vi "test-pose2d.vi"() -> ()   [LabVIEW 2019]
uses:
  <vilib>/Rock Robotics/WPI/ThirdParty/JAS_Junk/TrajLib/Translation_Equals.vi
  <vilib>/Rock Robotics/WPI/ThirdParty/JAS_Junk/TrajLib/Rotation_Equals.vi
  <vilib>/Rock Robotics/WPI/ThirdParty/JAS_Junk/TrajLib/Transform_Create_PosePose.vi
  <vilib>/Rock Robotics/WPI/ThirdParty/JAS_Junk/TrajLib/Pose_TransformBy.vi
  <vilib>/Rock Robotics/WPI/ThirdParty/JAS_Junk/TrajLib/Rotation_UnaryMinus.vi
  <vilib>/Rock Robotics/WPI/ThirdParty/JAS_Junk/TrajLib/Translation_RotateBy.vi
  <vilib>/Rock Robotics/WPI/ThirdParty/JAS_Junk/TrajLib/Translation_Minus.vi
  <vilib>/Rock Robotics/WPI/ThirdParty/JAS_Junk/TrajLib/Rotation_Minus.vi
  <vilib>/Rock Robotics/WPI/ThirdParty/JAS_Junk/TrajLib/Translation_Plus.vi
  <vilib>/Rock Robotics/WPI/ThirdParty/JAS_Junk/TrajLib/Rotation_Plus.vi
  <vilib>/Rock Robotics/WPI/ThirdParty/JAS_Junk/TrajLib/Rotation_RotateBy.vi
  <vilib>/Rock Robotics/WPI/ThirdParty/JAS_Junk/TrajLib/Rotation_CreateXY.vi
  <vilib>/Rock Robotics/WPI/ThirdParty/JAS_Junk/TrajLib/Util_CalcDist.vi
  <vilib>/Rock Robotics/WPI/ThirdParty/JAS_Junk/TrajLib/Trajectory_Library.lvlib
panel:
  out "T4 -- Deg -- 0":dbl
  out "T4 -- y -- 0":dbl
  out "T4 -- X -- 0":dbl
  out "T3 - False":bool
  out "T2 - True":bool
  out "T1 -- Deg -- 0":dbl
  out "T1 -- y -- 0":dbl
  out "T1 -- X -- 0":dbl
  out "T0 -- Deg -- 0":dbl
  out "T0 -- y -- 0":dbl
  out "T0 -- X -- 0":dbl
  # "Pose2D Test"
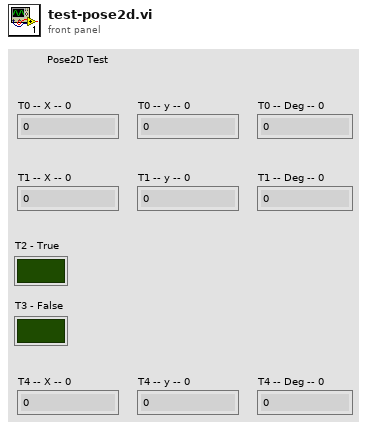
[diagram p1: front panel]
types:
  T1 = typedef "Trajectory_Library.lvlib/TRANSLATION2D.ctl" = cluster{"X":dbl, "Y":dbl}
  T2 = typedef "Trajectory_Library.lvlib/ROTATION2D.ctl" = cluster{"VALUE":dbl, "COS":dbl, "SIN":dbl}
  T3 = typedef "Trajectory_Library.lvlib/POSE2D.ctl" = cluster{"TRANSLATION":T1, "ROTATION":T2}
  T4 = typedef "Trajectory_Library.lvlib/TRANSFORM2D.ctl" = cluster{"TRANSLATION":T1, "ROTATION":T2}
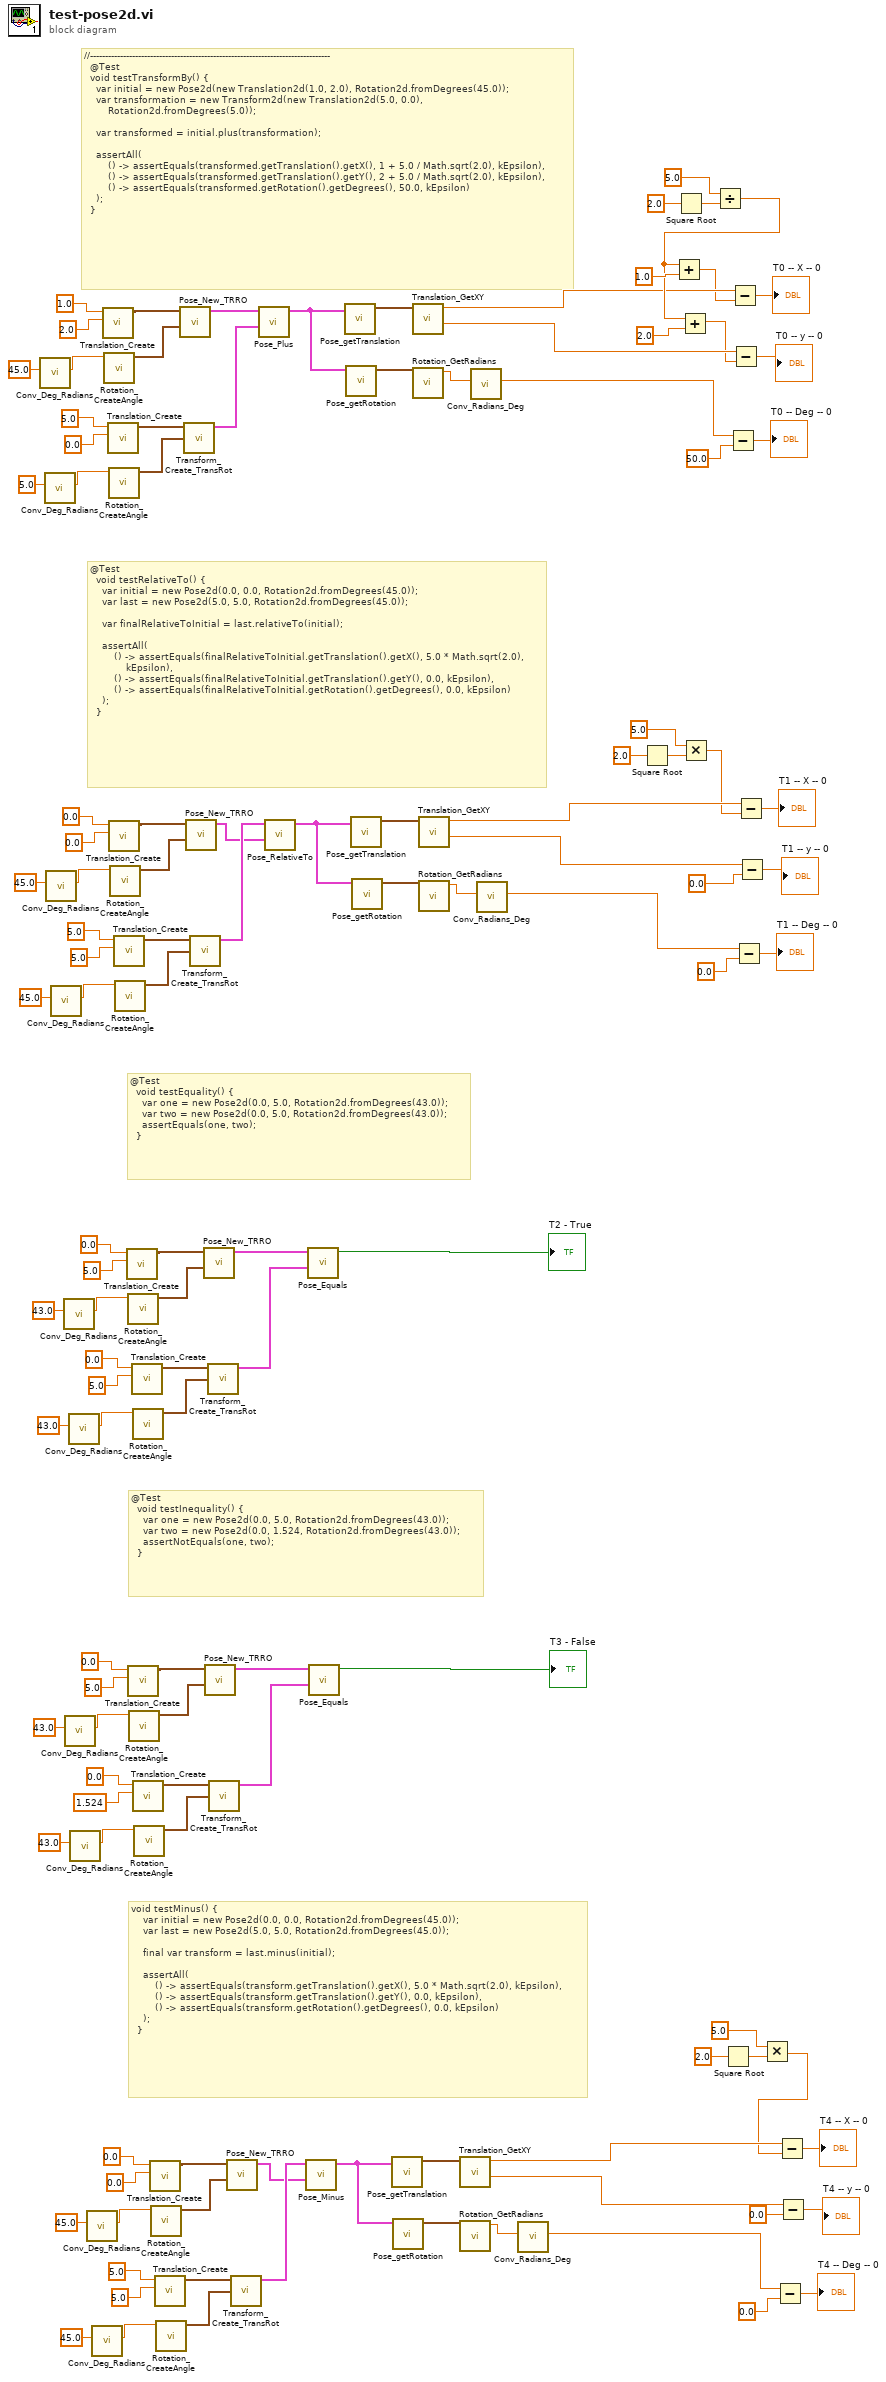
[diagram p0: block diagram]
diagram:
  # "void testMinus() {\n    var initial = new Pose2d(0.0, 0.0, Rotation2d.fromDegrees(45.0));\n    var last = new Pose2d(5.0, 5.0, Rotation2d.fromDegrees(45.0));\n\n    final var transform = last.minus(initial);\n\n    assertAll(\n        () -> assertEquals(transform.getTranslation().getX(), 5.0 * Math.sqrt(2.0), kEpsilon),\n        () -> assertEquals(transform.getTranslation().getY(), 0.0, kEpsilon),\n        () -> assertEquals(transform.getRotation().getDegrees(), 0.0, kEpsilon)\n    );\n  }"
  # "@Test\n  void testInequality() {\n    var one = new Pose2d(0.0, 5.0, Rotation2d.fromDegrees(43.0));\n    var two = new Pose2d(0.0, 1.524, Rotation2d.fromDegrees(43.0));\n    assertNotEquals(one, two);\n  }"
  # "@Test\n  void testEquality() {\n    var one = new Pose2d(0.0, 5.0, Rotation2d.fromDegrees(43.0));\n    var two = new Pose2d(0.0, 5.0, Rotation2d.fromDegrees(43.0));\n    assertEquals(one, two);\n  }"
  # "@Test\n  void testRelativeTo() {\n    var initial = new Pose2d(0.0, 0.0, Rotation2d.fromDegrees(45.0));\n    var last = new Pose2d(5.0, 5.0, Rotation2d.fromDegrees(45.0));\n\n    var finalRelativeToInitial = last.relativeTo(initial);\n\n    assertAll(\n        () -> assertEquals(finalRelativeToInitial.getTranslation().getX(), 5.0 * Math.sqrt(2.0),\n            kEpsilon),\n        () -> assertEquals(finalRelativeToInitial.getTranslation().getY(), 0.0, kEpsilon),\n        () -> assertEquals(finalRelativeToInitial.getRotation().getDegrees(), 0.0, kEpsilon)\n    );\n  }"
  # "//--------------------------------------------------------------------------------\n  @Test\n  void testTransformBy() {\n    var initial = new Pose2d(new Translation2d(1.0, 2.0), Rotation2d.fromDegrees(45.0));\n    var transformation = new Transform2d(new Translation2d(5.0, 0.0),\n        Rotation2d.fromDegrees(5.0));\n\n    var transformed = initial.plus(transformation);\n\n    assertAll(\n        () -> assertEquals(transformed.getTranslation().getX(), 1 + 5.0 / Math.sqrt(2.0), kEpsilon),\n        () -> assertEquals(transformed.getTranslation().getY(), 2 + 5.0 / Math.sqrt(2.0), kEpsilon),\n        () -> assertEquals(transformed.getRotation().getDegrees(), 50.0, kEpsilon)\n    );\n  }"
  n1 = call <vilib>:"Conv_Deg_Radians.vi"("Degress"=45.0) -> ("Radians"=w118:dbl)  [unwired: 10 in]
  n2 = call <vilib>:"Conv_Deg_Radians.vi"("Degress"=5.0) -> ("Radians"=w113:dbl)  [unwired: 10 in]
  n3 = call <vilib>:"Conv_Deg_Radians.vi"("Degress"=45.0) -> ("Radians"=w85:dbl)  [unwired: 10 in]
  n4 = call <vilib>:"Conv_Deg_Radians.vi"("Degress"=45.0) -> ("Radians"=w80:dbl)  [unwired: 10 in]
  n5 = call <vilib>:"Conv_Deg_Radians.vi"("Degress"=43.0) -> ("Radians"=w57:dbl)  [unwired: 10 in]
  n6 = call <vilib>:"Conv_Deg_Radians.vi"("Degress"=43.0) -> ("Radians"=w42:dbl)  [unwired: 10 in]
  n7 = call <vilib>:"Conv_Deg_Radians.vi"("Degress"=43.0) -> ("Radians"=w52:dbl)  [unwired: 10 in]
  n8 = call <vilib>:"Conv_Deg_Radians.vi"("Degress"=43.0) -> ("Radians"=w37:dbl)  [unwired: 10 in]
  n9 = call <vilib>:"Conv_Deg_Radians.vi"("Degress"=45.0) -> ("Radians"=w25:dbl)  [unwired: 10 in]
  n10 = call <vilib>:"Conv_Deg_Radians.vi"("Degress"=45.0) -> ("Radians"=w20:dbl)  [unwired: 10 in]
  n11 = call <vilib>:"Translation_Create.vi"("Y"=2.0, "X"=1.0) -> ("TRANSLATION"=w117:T1)  [unwired: 9 in]
  n12 = call <vilib>:"Rotation_CreateAngle.vi"("Angle"=w118) -> ("ROTATION"=w116:T2)  [unwired: 10 in]
  n13 = call <vilib>:"Translation_Create.vi"("Y"=0.0, "X"=5.0) -> ("TRANSLATION"=w111:T1)  [unwired: 9 in]
  n14 = call <vilib>:"Rotation_CreateAngle.vi"("Angle"=w113) -> ("ROTATION"=w110:T2)  [unwired: 10 in]
  n15 = call <vilib>:"Translation_Create.vi"("Y"=0.0, "X"=0.0) -> ("TRANSLATION"=w84:T1)  [unwired: 9 in]
  n16 = call <vilib>:"Rotation_CreateAngle.vi"("Angle"=w85) -> ("ROTATION"=w83:T2)  [unwired: 10 in]
  n17 = call <vilib>:"Translation_Create.vi"("Y"=5.0, "X"=5.0) -> ("TRANSLATION"=w78:T1)  [unwired: 9 in]
  n18 = call <vilib>:"Rotation_CreateAngle.vi"("Angle"=w80) -> ("ROTATION"=w77:T2)  [unwired: 10 in]
  n19 = call <vilib>:"Translation_Create.vi"("Y"=5.0, "X"=0.0) -> ("TRANSLATION"=w56:T1)  [unwired: 9 in]
  n20 = call <vilib>:"Rotation_CreateAngle.vi"("Angle"=w57) -> ("ROTATION"=w55:T2)  [unwired: 10 in]
  n21 = call <vilib>:"Translation_Create.vi"("Y"=5.0, "X"=0.0) -> ("TRANSLATION"=w41:T1)  [unwired: 9 in]
  n22 = call <vilib>:"Rotation_CreateAngle.vi"("Angle"=w42) -> ("ROTATION"=w40:T2)  [unwired: 10 in]
  n23 = call <vilib>:"Translation_Create.vi"("Y"=5.0, "X"=0.0) -> ("TRANSLATION"=w50:T1)  [unwired: 9 in]
  n24 = call <vilib>:"Rotation_CreateAngle.vi"("Angle"=w52) -> ("ROTATION"=w49:T2)  [unwired: 10 in]
  n25 = call <vilib>:"Translation_Create.vi"("Y"=1.524, "X"=0.0) -> ("TRANSLATION"=w35:T1)  [unwired: 9 in]
  n26 = call <vilib>:"Rotation_CreateAngle.vi"("Angle"=w37) -> ("ROTATION"=w34:T2)  [unwired: 10 in]
  n27 = call <vilib>:"Translation_Create.vi"("Y"=0.0, "X"=0.0) -> ("TRANSLATION"=w24:T1)  [unwired: 9 in]
  n28 = call <vilib>:"Rotation_CreateAngle.vi"("Angle"=w25) -> ("ROTATION"=w23:T2)  [unwired: 10 in]
  n29 = call <vilib>:"Translation_Create.vi"("Y"=5.0, "X"=5.0) -> ("TRANSLATION"=w18:T1)  [unwired: 9 in]
  n30 = call <vilib>:"Rotation_CreateAngle.vi"("Angle"=w20) -> ("ROTATION"=w17:T2)  [unwired: 10 in]
  n31 = call <vilib>:"Pose_New_TRRO.vi"("ROTATION"=w116, "TRANSLATION"=w117) -> ("outPOSE"=w109:T3)  [unwired: 9 in]
  n32 = call <vilib>:"Transform_Create_TransRot.vi"("ROTATION"=w110, "TRANSLATION"=w111) -> ("TRANSFORM"=w108:T4)  [unwired: 9 in]
  n33 = call <vilib>:"Pose_New_TRRO.vi"("ROTATION"=w83, "TRANSLATION"=w84) -> ("outPOSE"=w62:T3)  [unwired: 9 in]
  n34 = call <vilib>:"Transform_Create_TransRot.vi"("ROTATION"=w77, "TRANSLATION"=w78) -> ("TRANSFORM"=w63:T4)  [unwired: 9 in]
  n35 = call <vilib>:"Pose_New_TRRO.vi"("ROTATION"=w55, "TRANSLATION"=w56) -> ("outPOSE"=w48:T3)  [unwired: 9 in]
  n36 = call <vilib>:"Pose_New_TRRO.vi"("ROTATION"=w40, "TRANSLATION"=w41) -> ("outPOSE"=w33:T3)  [unwired: 9 in]
  n37 = call <vilib>:"Transform_Create_TransRot.vi"("ROTATION"=w49, "TRANSLATION"=w50) -> ("TRANSFORM"=w47:T4)  [unwired: 9 in]
  n38 = call <vilib>:"Transform_Create_TransRot.vi"("ROTATION"=w34, "TRANSLATION"=w35) -> ("TRANSFORM"=w32:T4)  [unwired: 9 in]
  n39 = call <vilib>:"Pose_New_TRRO.vi"("ROTATION"=w23, "TRANSLATION"=w24) -> ("outPOSE"=w3:T3)  [unwired: 9 in]
  n40 = call <vilib>:"Transform_Create_TransRot.vi"("ROTATION"=w17, "TRANSLATION"=w18) -> ("TRANSFORM"=w4:T4)  [unwired: 9 in]
  n41 = call <vilib>:"Pose_Plus.vi"("other TRANSFORM"=w108, "in POSE"=w109) -> ("out POSE"=w106:T3)  [unwired: 9 in]
  n42 = call <vilib>:"Pose_RelativeTo.vi"("other POSE"=w62, "in POSE"=w63) -> ("out POSE"=w75:T3)  [unwired: 9 in]
  n43 = call <vilib>:"Pose_Minus.vi"("other TRANSFORM"=w3, "in POSE"=w4) -> ("outTRANSFORM"=w15:T4)  [unwired: 9 in]
  n44 = call <vilib>:"Pose_Equals.vi"("other POSE"=w47, "in POSE"=w48) -> ("Equals"=→"T2 - True":bool)  [unwired: 9 in]
  n45 = call <vilib>:"Pose_Equals.vi"("other POSE"=w32, "in POSE"=w33) -> ("Equals"=→"T3 - False":bool)  [unwired: 9 in]
  n46 = call <vilib>:"Pose_getTranslation.vi"("in POSE"=w106) -> ("outTRANSLATION"=w107:T1)  [unwired: 10 in]
  n47 = call <vilib>:"Pose_getRotation.vi"("in POSE"=w106) -> ("out ROTATION"=w105:T2)  [unwired: 10 in]
  n48 = call <vilib>:"Pose_getTranslation.vi"("in POSE"=w75) -> ("outTRANSLATION"=w76:T1)  [unwired: 10 in]
  n49 = call <vilib>:"Pose_getRotation.vi"("in POSE"=w75) -> ("out ROTATION"=w74:T2)  [unwired: 10 in]
  n50 = call <vilib>:"Pose_getTranslation.vi"("in POSE"=w15) -> ("outTRANSLATION"=w16:T1)  [unwired: 10 in]
  n51 = call <vilib>:"Pose_getRotation.vi"("in POSE"=w15) -> ("out ROTATION"=w14:T2)  [unwired: 10 in]
  n52 = call <vilib>:"Translation_GetXY.vi"("In Translation"=w107) -> ("Y"=w95:dbl, "X"=w96:dbl)  [unwired: 9 in]
  n53 = call <vilib>:"Rotation_GetRadians.vi"("in ROTATION"=w105) -> ("AngleRadians"=w104:dbl)  [unwired: 10 in]
  n54 = call <vilib>:"Translation_GetXY.vi"("In Translation"=w76) -> ("Y"=w67:dbl, "X"=w68:dbl)  [unwired: 9 in]
  n55 = call <vilib>:"Rotation_GetRadians.vi"("in ROTATION"=w74) -> ("AngleRadians"=w73:dbl)  [unwired: 10 in]
  n56 = call <vilib>:"Translation_GetXY.vi"("In Translation"=w16) -> ("Y"=w7:dbl, "X"=w8:dbl)  [unwired: 9 in]
  n57 = call <vilib>:"Rotation_GetRadians.vi"("in ROTATION"=w14) -> ("AngleRadians"=w13:dbl)  [unwired: 10 in]
  n58 = call <vilib>:"Conv_Radians_Deg.vi"("Radians"=w104) -> ("Degrees"=w91:dbl)  [unwired: 10 in]
  n59 = call <vilib>:"Conv_Radians_Deg.vi"("Radians"=w73) -> ("Degrees"=w65:dbl)  [unwired: 10 in]
  n60 = call <vilib>:"Conv_Radians_Deg.vi"("Radians"=w13) -> ("Degrees"=w5:dbl)  [unwired: 10 in]
  n61 = Square Root(x=2.0) -> (sqrt(x)=w71:dbl)
  n62 = Square Root(x=2.0) -> (sqrt(x)=w102:dbl)
  n63 = Multiply(x=5.0, y=w71) -> (x*y=w61:dbl)
  n64 = Divide(x=5.0, y=w102) -> (x/y=w98:dbl)
  n65 = Add(x=w98, y=1.0) -> (x+y=w93:dbl)
  n66 = Add(x=w98, y=2.0) -> (x+y=w94:dbl)
  n67 = Square Root(x=2.0) -> (sqrt(x)=w11:dbl)
  n68 = Subtract(x=w91, y=50.0) -> (x-y=→"T0 -- Deg -- 0":dbl)
  n69 = Subtract(x=w96, y=w93) -> (x-y=→"T0 -- X -- 0":dbl)
  n70 = Subtract(x=w95, y=w94) -> (x-y=→"T0 -- y -- 0":dbl)
  n71 = Subtract(x=w65, y=0.0) -> (x-y=→"T1 -- Deg -- 0":dbl)
  n72 = Subtract(x=w68, y=w61) -> (x-y=→"T1 -- X -- 0":dbl)
  n73 = Subtract(x=w67, y=0.0) -> (x-y=→"T1 -- y -- 0":dbl)
  n74 = Multiply(x=5.0, y=w11) -> (x*y=w2:dbl)
  n75 = Subtract(x=w5, y=0.0) -> (x-y=→"T4 -- Deg -- 0":dbl)
  n76 = Subtract(x=w8, y=w2) -> (x-y=→"T4 -- X -- 0":dbl)
  n77 = Subtract(x=w7, y=0.0) -> (x-y=→"T4 -- y -- 0":dbl)
